vi "Object Factory Dynamic Dispatch.vi"(6 "Cluster Component":bool, 8 "error in (no error)":errorcluster, 11 "GOject In":refnum<vi>) -> (0 "error out":errorcluster, 1 "Is Visible":bool, 2 "Is Control":bool, 3 "Object Out":refnum<class "Object.lvclass">, 4 "All Objects Created":refnum<class "Object.lvclass">[](array[class]), 5 "Is Indicator":bool)   [LabVIEW 2017, in "Front Panel Publisher.lvlib" / "Web Front Panel.lvclass"]
doc: "Convert FP refs into \"HTML\" objects"
uses:
  Web Front Panel.lvclass
  Front Panel Objects/Select_class/Select.lvclass
  Front Panel Objects/Progressbar_class/Progressbar.lvclass
  Front Panel Objects/Text_class/Text.lvclass
  Front Panel Objects/Object_class/Object.lvclass
  Front Panel Objects/Control_class/Control.lvclass
  Front Panel Objects/Numeric_class/Numeric.lvclass
  Front Panel Objects/String_class/String.lvclass
  Front Panel Objects/Boolean_class/Boolean.lvclass
  Front Panel Objects/Graph_class/Graph.lvclass
  Front Panel Objects/Cluster_class/Front Panel Objects/String_class/Cluster.lvclass
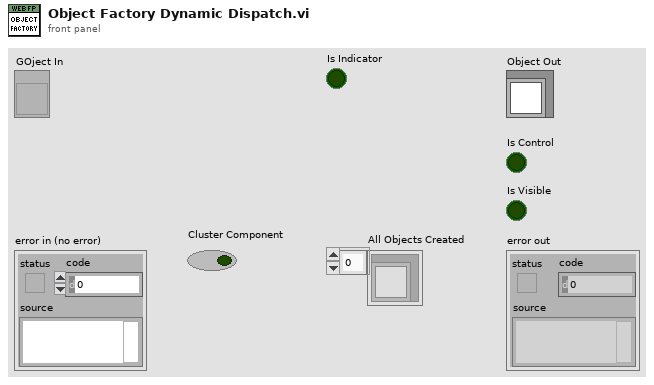
[diagram p1: front panel]
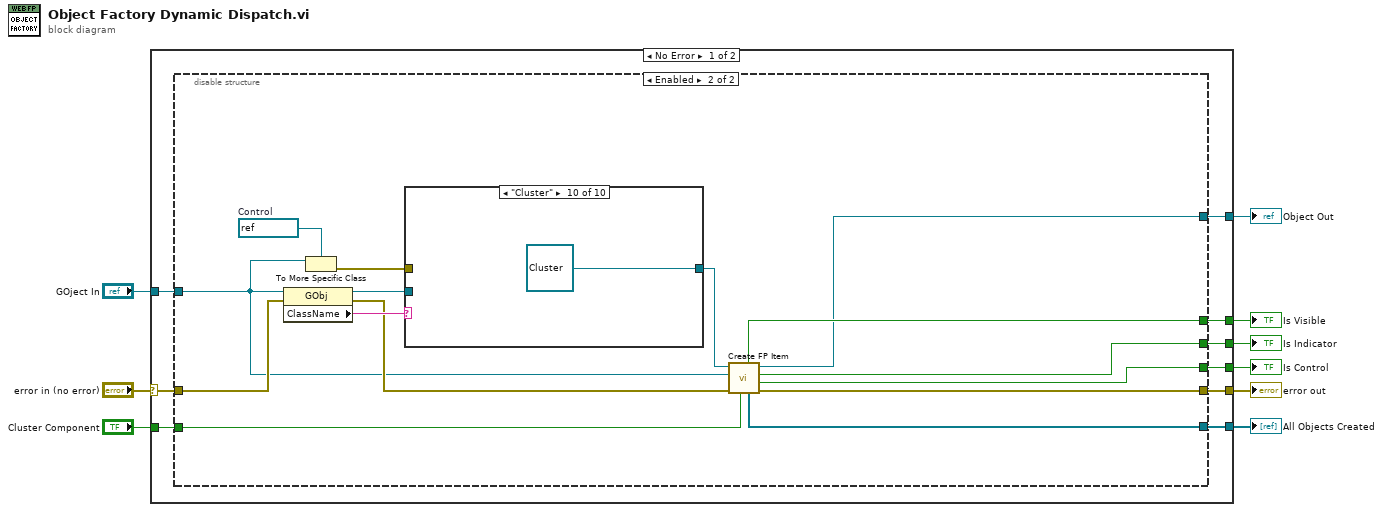
[diagram p0: block diagram]
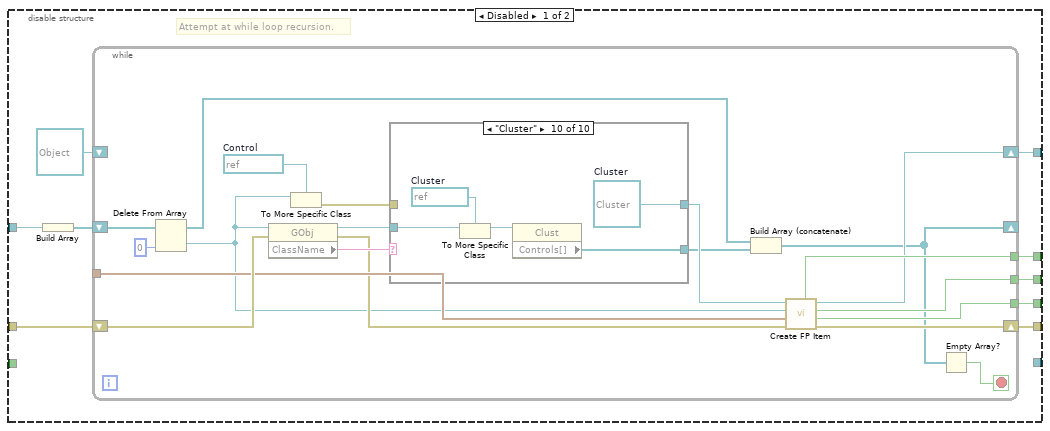
[diagram p2: hidden frame]
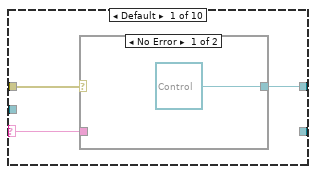
[diagram p3: hidden frame]
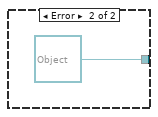
[diagram p4: hidden frame]
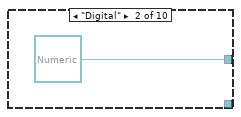
[diagram p5: hidden frame]
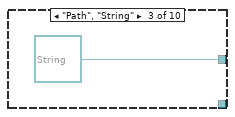
[diagram p6: hidden frame]
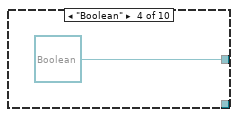
[diagram p7: hidden frame]
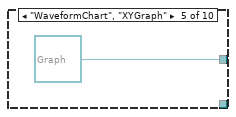
[diagram p8: hidden frame]
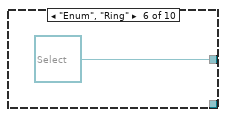
[diagram p9: hidden frame]
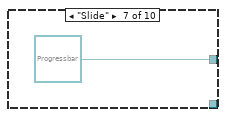
[diagram p10: hidden frame]
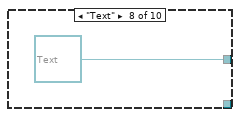
[diagram p11: hidden frame]
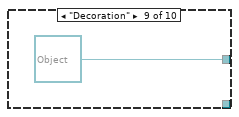
[diagram p12: hidden frame]
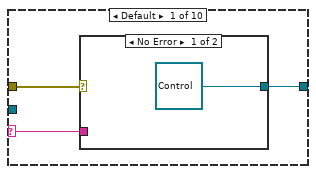
[diagram p13: hidden frame]
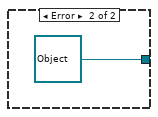
[diagram p14: hidden frame]
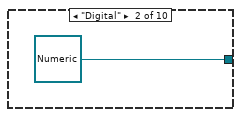
[diagram p15: hidden frame]
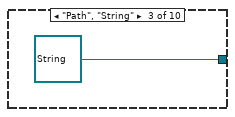
[diagram p16: hidden frame]
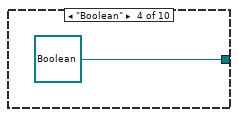
[diagram p17: hidden frame]
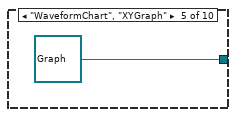
[diagram p18: hidden frame]
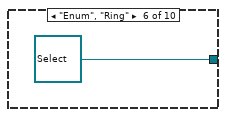
[diagram p19: hidden frame]
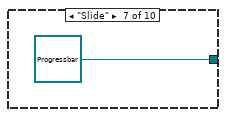
[diagram p20: hidden frame]
diagram:
  n1 = case shown="No Error" "error in (no error)" {
    selector: "error in (no error)" -> [w18 w96]
    tunnel: [w12 w96] -> w8
    tunnel: "GOject In" -> [w17 _]
    tunnel: [w16 _] -> w6
    tunnel: [w15 _] -> w5
    tunnel: [w14 _] -> w4
    tunnel: [w13 _] -> w3
    tunnel: [w11 _] -> w2
    tunnel: "Cluster Component" -> [w10 _]
    frame No Error {
      n2 = disable-structure shown="Enabled" {
        disable-tunnel: w18 -> [w28 w81]
        disable-tunnel: w17 -> [w27 w71]
        disable-tunnel: [w25 w80] -> w16
        disable-tunnel: [w24 w79] -> w15
        disable-tunnel: [w23 w78] -> w14
        disable-tunnel: [w22 w68] -> w13
        disable-tunnel: [w21 w67] -> w12
        disable-tunnel: [_ w70] -> w11
        disable-tunnel: w10 -> [_ w69]
        frame Disabled {
          # "Attempt at while loop recursion."
          n3 = Build Array(w27) -> (w20:refnum<vi>[])
          n4 = while {
            tunnel: [w47] -> w26
            tunnel: [w46] -> w25
            tunnel: [w45] -> w24
            tunnel: [w44] -> w23
            shift-right: [w37] -> w21
            shift-left: w28 -> [w48]
            shift-right: [w30] -> _
            shift-left: w20 -> [w34]
            shift-right: [w39] -> w22
            shift-left: refnum<class "Object.lvclass"> refnum ("GObject out") -> [_]
            stop <- w29 stop-if-true
            w42 = refnum<vi> refnum  # Control
            n5 = Delete From Array(array=w34, index=0) -> (deleted portion=w35:refnum<vi>, array with subset deleted=w31:refnum<vi>[])  [unwired: 1 in]
            n6 = property class="GObj"(reference=w35, error in=w48) -> (reference out=w33:refnum<vi>, error out=w38:errorcluster, "ClassName"=w43:string)
            n7 = To More Specific Class(target class=w42, reference=w35) -> (error out=w41:errorcluster)  [unwired: 1 in, 1 out]
            n8 = case shown="\"Cluster\"" w43 {
              selector: w43 -> [w50 _ _ _ _ _ _ _ _ _]
              tunnel: w41 -> [w51 _ _ _ _ _ _ _ _ _]
              tunnel: [w49 refnum<class "Numeric.lvclass"> refnum ("Front Panel Publisher.lvlib:Control") refnum<class "String.lvclass"> refnum ("Front Panel Publisher.lvlib:Control") refnum<class "Boolean.lvclass"> refnum ("Front Panel Publisher.lvlib:BooleanControl") refnum<class "Graph.lvclass"> refnum ("Front Panel Publisher.lvlib:Control") refnum<class "Select.lvclass"> refnum ("Front Panel Publisher.lvlib:Control") refnum<class "Progressbar.lvclass"> refnum ("Front Panel Publisher.lvlib:Control") refnum<class "Text.lvclass"> refnum ("Front Panel Publisher.lvlib:Text") refnum<class "Object.lvclass"> refnum ("Front Panel Publisher.lvlib:GObject") w66] -> w40
              tunnel: w33 -> [_ _ _ _ _ _ _ _ _ w65]
              tunnel: [_ _ _ _ _ _ _ _ _ w62] -> w32
              frame Default {
                n9 = case shown="No Error" w51 {
                  tunnel: w50 -> [_ _]
                  tunnel: [refnum<class "Control.lvclass"> refnum ("Front Panel Publisher.lvlib:Control") refnum<class "Object.lvclass"> refnum ("Front Panel Publisher.lvlib:GObject")] -> w49
                  frame No Error {
                  }
                  frame Error {
                  }
                }
              }
              frame "Digital" {
              }
              frame "Path", "String" {
              }
              frame "Boolean" {
              }
              frame "WaveformChart", "XYGraph" {
              }
              frame "Enum", "Ring" {
              }
              frame "Slide" {
              }
              frame "Text" {
              }
              frame "Decoration" {
              }
              frame "Cluster" {
                w63 = refnum<vi> refnum  # Cluster
                w66 = refnum<class "Cluster.lvclass"> refnum  # Cluster
                n10 = To More Specific Class(target class=w63, reference=w65) -> (specific class reference=w64:refnum<vi>)  [unwired: 1 in, 1 out]
                n11 = property class="Clust"(reference=w64) -> ("Controls[]"=w62:refnum<vi>[])  [unwired: 1 in, 2 out]
              }
            }
            n12 = Build Array (concatenate)(w31, w32) -> (w30:refnum<vi>[])
            n13 = call-dynamic "Create FP Item.vi"("error in (no error)"=w38, 9:w47, "GObject In"=w35, "GObject in"=w40) -> ("error out"=w37:errorcluster, "Is Control"=w45:bool, "Is Indicator"=w46:bool, "GObject out"=w39:refnum<class "Object.lvclass">, "Is Visible"=w44:bool)  [unwired: 2 in, 1 out]
            n14 = Empty Array?(array=w30) -> (empty?=w29:bool)
          }
        }
        frame Enabled {
          w76 = refnum<vi> refnum  # Control
          n15 = property class="GObj"(reference=w71, error in=w81) -> (reference out=w72:refnum<vi>, error out=w73:errorcluster, "ClassName"=w77:string)
          n16 = To More Specific Class(target class=w76, reference=w71) -> (error out=w75:errorcluster)  [unwired: 1 in, 1 out]
          n17 = case shown="\"Cluster\"" w77 {
            selector: w77 -> [w83 _ _ _ _ _ _ _ _ _]
            tunnel: w75 -> [w84 _ _ _ _ _ _ _ _ _]
            tunnel: [w82 refnum<class "Numeric.lvclass"> refnum ("Front Panel Publisher.lvlib:Control") refnum<class "String.lvclass"> refnum ("Front Panel Publisher.lvlib:Control") refnum<class "Boolean.lvclass"> refnum ("Front Panel Publisher.lvlib:BooleanControl") refnum<class "Graph.lvclass"> refnum ("Front Panel Publisher.lvlib:Control") refnum<class "Select.lvclass"> refnum ("Front Panel Publisher.lvlib:Control") refnum<class "Progressbar.lvclass"> refnum ("Front Panel Publisher.lvlib:Control") refnum<class "Text.lvclass"> refnum ("Front Panel Publisher.lvlib:Text") refnum<class "Object.lvclass"> refnum ("Front Panel Publisher.lvlib:GObject") refnum<class "Cluster.lvclass"> refnum ("Cluster")] -> w74
            tunnel: w72 -> [_ _ _ _ _ _ _ _ _ _]
            frame Default {
              n18 = case shown="No Error" w84 {
                tunnel: w83 -> [_ _]
                tunnel: [refnum<class "Control.lvclass"> refnum ("Front Panel Publisher.lvlib:Control") refnum<class "Object.lvclass"> refnum ("Front Panel Publisher.lvlib:GObject")] -> w82
                frame No Error {
                }
                frame Error {
                }
              }
            }
            frame "Digital" {
            }
            frame "Path", "String" {
            }
            frame "Boolean" {
            }
            frame "WaveformChart", "XYGraph" {
            }
            frame "Enum", "Ring" {
            }
            frame "Slide" {
            }
            frame "Text" {
            }
            frame "Decoration" {
            }
            frame "Cluster" {
            }
          }
          n19 = call-dynamic "Create FP Item.vi"("Cluster Component"=w69, "error in (no error)"=w73, "GObject In"=w71, "GObject in"=w74) -> ("error out"=w67:errorcluster, "Is Control"=w79:bool, "Is Indicator"=w80:bool, "GObject out"=w68:refnum<class "Object.lvclass">, "All Objects Created"=w70:refnum<class "Object.lvclass">[], "Is Visible"=w78:bool)  [unwired: 2 in]
        }
      }
    }
    frame Error {
    }
  }
  "error out" <- w8
  "Object Out" <- w3
  "Is Indicator" <- w6
  "Is Control" <- w5
  "Is Visible" <- w4
  "All Objects Created" <- w2
